vi "Voltage K230 Coarse.vi"() -> ()   [LabVIEW 2020]
panel:
  out "Voltage K230 Coarse":dbl
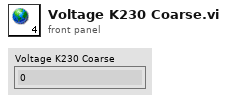
[diagram p1: front panel]
diagram:
